vi "Format Connection String.vi"(8 "error in":errorcluster, 11 "Connection Information":T1) -> (0 "error out":errorcluster, 3 "connection string":string)   [LabVIEW 2016, in "PQ Support.lvlib"]
uses:
  Connection Information.ctl
  PQ Support.lvlib
  Connection/PQ Connection.lvclass
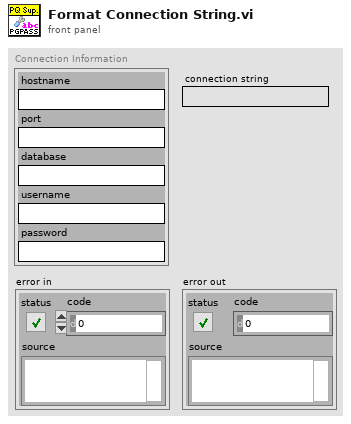
[diagram p1: front panel]
types:
  T1 = typedef "PQ Connection.lvclass/Connection Information.ctl" = cluster{"hostname":string, "port":string, "database":string, "username":string, "password":string}
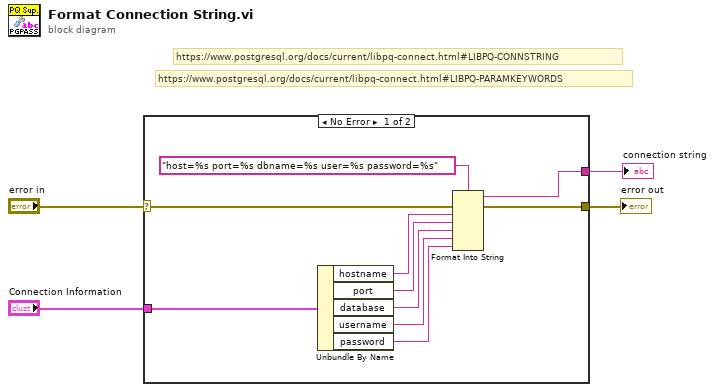
[diagram p0: block diagram]
diagram:
  # "https://www.postgresql.org/docs/current/libpq-connect.html#LIBPQ-PARAMKEYWORDS"
  # "https://www.postgresql.org/docs/current/libpq-connect.html#LIBPQ-CONNSTRING"
  n1 = case shown="No Error" "error in" {
    selector: "error in" -> [w5 w15]
    tunnel: "Connection Information" -> [w13 _]
    tunnel: [w7 _] -> w3
    tunnel: [w6 w15] -> w2
    frame No Error {
      n2 = Unbundle By Name(w13) -> ("hostname"=w12:string, "port"=w11:string, "database"=w10:string, "username"=w9:string, "password"=w8:string)
      n3 = Format Into String(format string="host=%s port=%s dbname=%s user=%s password=%s", error in=w5, w12, w11, w10, w9, w8) -> (resulting string=w7:string, error out=w6:errorcluster)  [unwired: 1 in]
    }
    frame Error {
    }
  }
  "connection string" <- w3
  "error out" <- w2
